vi "FPGA_VI.vi"() -> ()   [LabVIEW 2021]
uses:
  <vilib>/rvi/Emulation/niFpgaGetClockAttributes.vi
  <vilib>/rvi/Emulation/niFpgaSctlEmulationGetInTimedLoop.vi
  <vilib>/rvi/Emulation/niFpgaEmulationReportErrorSimple.vi
  <vilib>/rvi/eio/common/nirviEmuTemplateMethod_errors.vi
  <vilib>/rvi/interface/RandomDataEmulation/niFpgaRandomDataHandleErrors.vi
  <vilib>/rvi/Emulation/niFpgaCriticalErrorInLSC.vi
  <vilib>/eio/EIONode/EIONode.xnode
  <vilib>/rvi/DataTransferAndStorage/Container/XNode/niFpgaContainer.xnode
  <vilib>/rvi/interface/RandomDataEmulation/nirviRandomDataFpgaReadWriteTemplate.vi
panel:
  out "UserSwitch3:0_array":bool[](array[boolean])
  out "UserSwitch3":bool
  out "User Switch2":bool
  in  "UserLED3":bool
  in  "UserLED2":bool
  in  "UserLED1":bool
  in  "UserLED0":bool
  out "UserSwitch3:0":u8
  out "UserSwitch1":bool
  out "UserSwitch0":bool
  in  "Wait (mSec)":u32=200
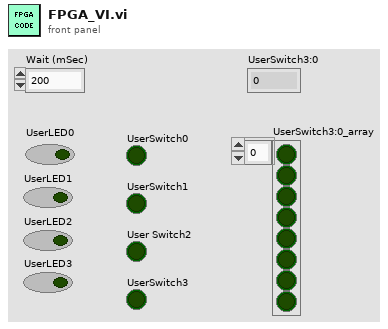
[diagram p1: front panel]
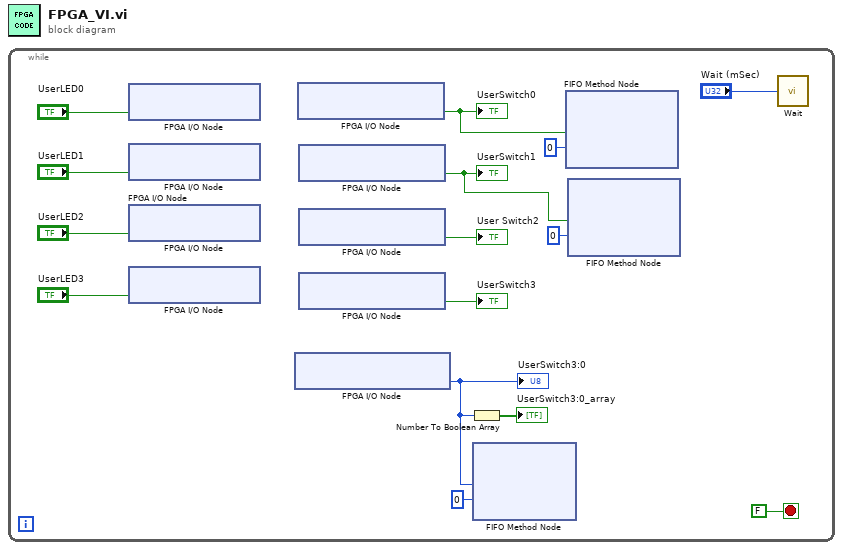
[diagram p0: block diagram]
diagram:
  n1 = while {
    stop <- FALSE stop-if-true
    n2 = xnode "FPGA I/O Node"("Mod7/User LED0"="UserLED0") -> ()  [unwired: 1 in, 1 out]
    n3 = xnode "FPGA I/O Node"("Mod7/User LED1"="UserLED1") -> ()  [unwired: 1 in, 1 out]
    n4 = xnode "FPGA I/O Node"("Mod7/User LED2"="UserLED2") -> ()  [unwired: 1 in, 1 out]
    n5 = xnode "FPGA I/O Node"() -> ()  [unwired: 1 in, 2 out]
    n6 = xnode "FPGA I/O Node"("Mod7/User LED3"="UserLED3") -> ()  [unwired: 1 in, 1 out]
    n7 = xnode "FPGA I/O Node"() -> ("Mod7/User Switch3:0"=w6:u8)  [unwired: 1 in, 1 out]
    "UserSwitch3:0" <- w6
    n8 = xnode "FPGA I/O Node"() -> ("Mod7/User Switch0"=w5:bool)  [unwired: 1 in, 1 out]
    "UserSwitch0" <- w5
    n9 = xnode "FPGA I/O Node"() -> ("Mod7/User Switch1"=w4:bool)  [unwired: 1 in, 1 out]
    "UserSwitch1" <- w4
    n10 = xnode "FPGA I/O Node"() -> ("Mod7/User Switch2"=→"User Switch2":bool)  [unwired: 1 in, 1 out]
    n11 = xnode "FPGA I/O Node"() -> ("Mod7/User Switch3"=→"UserSwitch3":bool)  [unwired: 1 in, 1 out]
    n12 = Number To Boolean Array(number=w6) -> (Boolean array=→"UserSwitch3:0_array":bool[])
    n13 = xnode ("FIFO Method Node")("Element"=w6, "Timeout"=0) -> ()  [unwired: 1 in, 2 out]
    n14 = xnode ("FIFO Method Node")("Element"=w5, "Timeout"=0) -> ()  [unwired: 1 in, 2 out]
    n15 = xnode ("FIFO Method Node")("Element"=w4, "Timeout"=0) -> ()  [unwired: 1 in, 2 out]
    n16 = call "Wait"("Count(mSec)"="Wait (mSec)") -> ()  [unwired: 1 out]
  }
